vi "Process.vi"(7 "SubPnl Refnum":refnum<vi>, 8 "error in (no error)":errorcluster, 9 "Payload":string, 10 "Command":string, 11 "Core Class":refnum<class>) -> (0 "error out":errorcluster, 2 "Response":string, 3 "Match Present?":bool)   [LabVIEW 2019, in "MicronTemplateService.lvlib"]
uses:
  MicronTemplateService.lvlib
  <vilib>/LabJSON/Typedefs/Settings.ctl
  4e70540b-6f8f-44f3-a0e1-83e2859abde4.vi
  0b93bba3-7b7b-446a-8943-9293762f4055.vi
  2355c958-d1c3-4277-9a8a-c12bb77dc7b9.vi
  <vilib>/LabJSON/APIs/RunVIRefnum.vi
  <vilib>/JDP Science/JSONtext/Variant to JSON Text.vi
  <vilib>/JDP Science/JSONtext/support/Format JSON Object.vi
  <vilib>/JDP Science/JSONtext/LVClass Serializer/JSONtext LVClass Serializer.lvclass
  <vilib>/LabJSON/LabJSON.lvlib
  <vilib>/JDP Science/JSONtext/JSONtext.lvlib
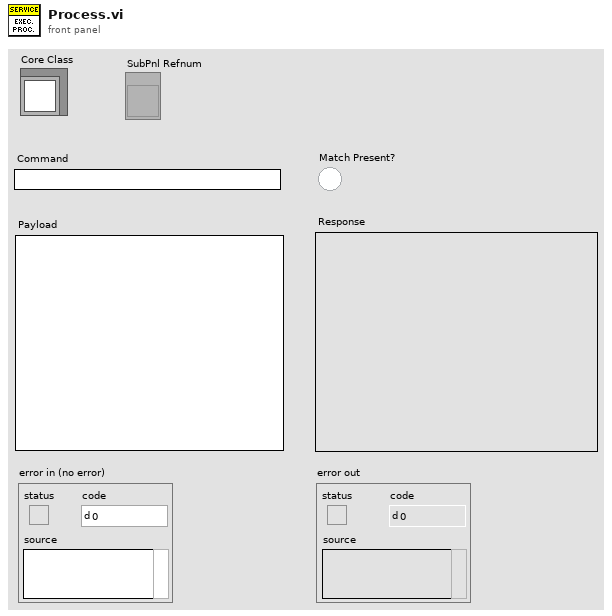
[diagram p1: front panel]
types:
  T1 = typedef "LabJSON.lvlib/Settings.ctl" = cluster{"Reinitialize to Default?":bool, "Show Front Panel?":bool, "Close Front Panel?":bool}
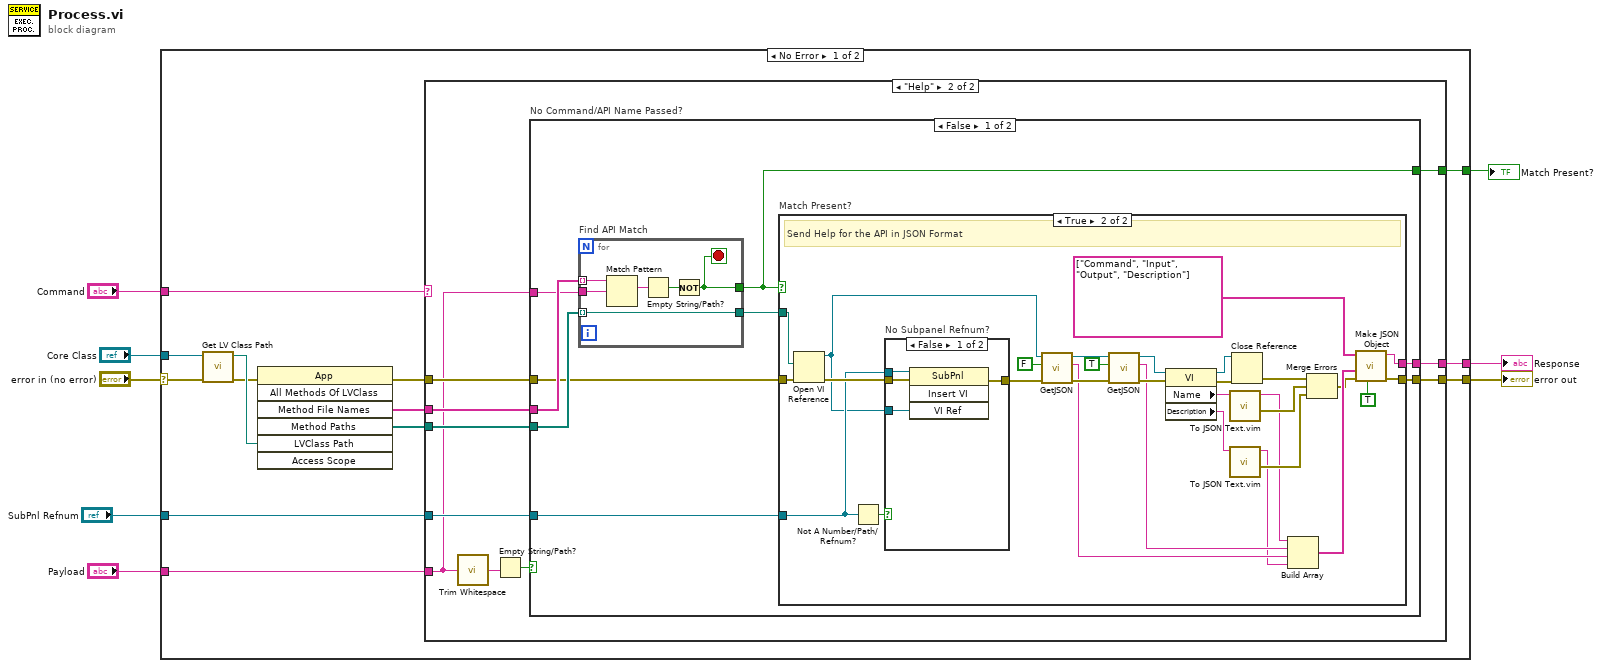
[diagram p0: block diagram]
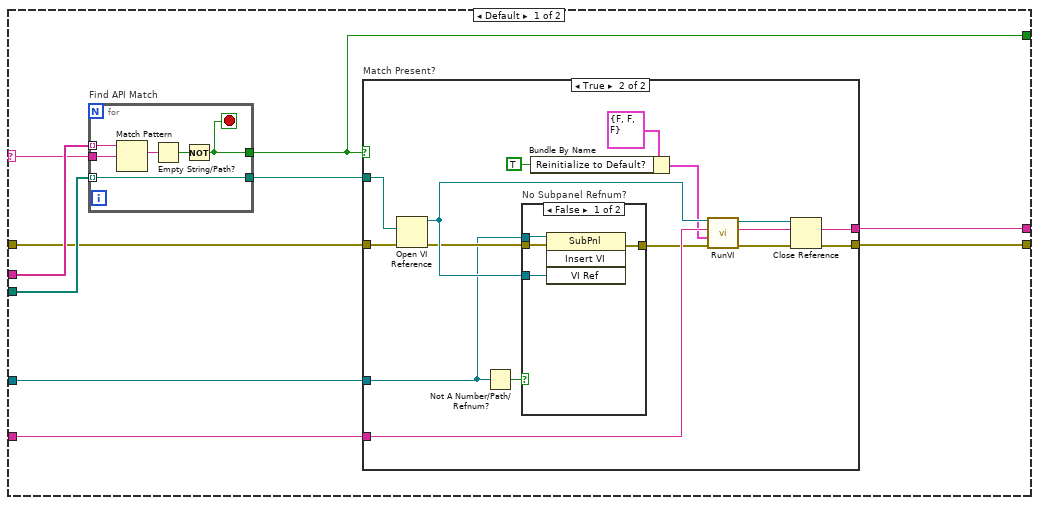
[diagram p2: hidden frame]
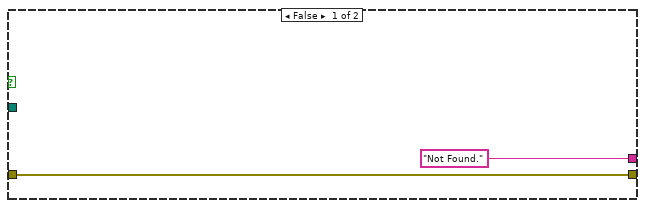
[diagram p5: hidden frame]
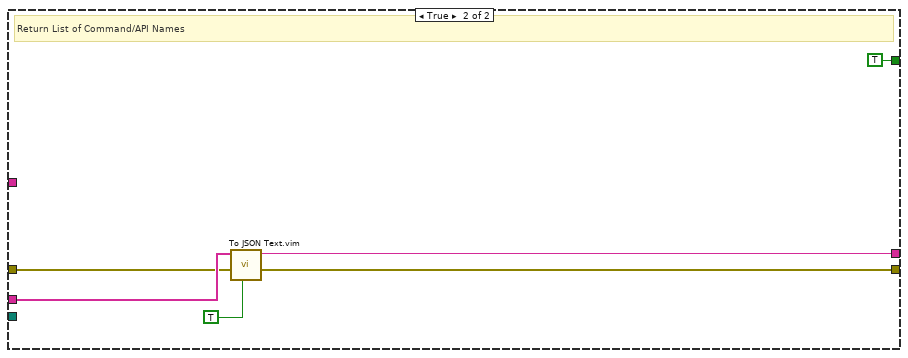
[diagram p7: hidden frame]
diagram:
  n1 = case shown="No Error" "error in (no error)" {
    selector: "error in (no error)" -> [w11 w127]
    tunnel: "Core Class" -> [w21 _]
    tunnel: "Command" -> [w17 _]
    tunnel: "Payload" -> [w16 _]
    tunnel: [w15 _] -> w5
    tunnel: "SubPnl Refnum" -> [w14 _]
    tunnel: [w10 w127] -> w2
    tunnel: [w9 _] -> w1
    frame No Error {
      n2 = call <vilib>:"Get LV Class Path.vi"("error in (no error)"=w11, "object"=w21) -> ("error out"=w13:errorcluster, "class path"=w20:path)  [unwired: 8 in]
      n3 = invoke class="App" method="All Methods Of LVClass"(error in=w13, "LVClass Path"=w20) -> (error out=w12:errorcluster, "Method File Names"=w19:string[], "Method Paths"=w18:path[])  [unwired: 5 in, 4 out]
      n4 = case shown="\"Help\"" w17 {
        selector: w17 -> [w29 _]
        tunnel: w19 -> [w31 w68]
        tunnel: w18 -> [w30 w67]
        tunnel: w16 -> [w28 w61]
        tunnel: [w27 w66] -> w15
        tunnel: w14 -> [w25 w65]
        tunnel: w12 -> [w24 w64]
        tunnel: [w23 w63] -> w10
        tunnel: [w22 w62] -> w9
        frame Default {
          n5 = for "Find API Match" {
            tunnel: w31 -> [w58] mode=indexing
            tunnel: w30 -> [w54] mode=indexing
            tunnel: w29 -> [w57]
            tunnel: [w54] -> w26
            tunnel: [w53] -> w22
            stop <- w53 stop-if-true
            n6 = Match Pattern(string=w58, regular expression=w57) -> (match substring=w56:string)  [unwired: 1 in, 3 out]
            n7 = Empty String/Path?(string/path=w56) -> (empty?=w55:bool)
            n8 = Not(x=w55) -> (.not. x?=w53:bool)
          }
          n9 = case "Match Present?" shown="True" w22 {
            tunnel: w28 -> [_ w47]
            tunnel: [_ w46] -> w27
            tunnel: w26 -> [_ w45]
            tunnel: w25 -> [_ w36]
            tunnel: w24 -> [w32 w40]
            tunnel: [w32 w34] -> w23
            frame False {
            }
            frame True {
              n10 = Open VI Reference(vi path=w45, error in (no error)=w40) -> (vi reference=w44:refnum<vi>, error out=w39:errorcluster)  [unwired: 4 in]
              n11 = Not A Number/Path/Refnum?(number/path/refnum=w36) -> (NaN/Path/Refnum?=w35:bool)
              n12 = case "No Subpanel Refnum?" shown="False" w35 {
                tunnel: w44 -> [w51 _]
                tunnel: w39 -> [w50 w52]
                tunnel: [w49 w52] -> w38
                tunnel: w36 -> [w48 _]
                frame False {
                  n13 = invoke class="SubPnl" method="Insert VI"(reference=w48, error in=w50, "VI Ref"=w51) -> (error out=w49:errorcluster)  [unwired: 1 in, 3 out]
                }
                frame True {
                }
              }
              n14 = Bundle By Name(cluster=T1 {"Reinitialize to Default?"=FALSE, "Show Front Panel?"=FALSE, "Close Front Panel?"=FALSE} ("Settings"), "Reinitialize to Default?"=TRUE) -> (w42:T1)
              n15 = call-poly <vilib>:"RunVI.vi"("Error In"=w38, "Settings"=w42, "JSON Input"=w47, "VI Refnum In"=w44) -> ("Error Out"=w37:errorcluster, "JSON Output"=w46:string, "VI Refnum Out"=w33:refnum<vi>)  [unwired: 5 in]
              n16 = Close Reference(reference=w33, error in (no error)=w37) -> (error out=w34:errorcluster)
            }
          }
        }
        frame "Help" {
          n17 = call <vilib>:"Trim Whitespace.vi"("string"=w61) -> ("trimmed string"=w60:string)  [unwired: 1 in]
          n18 = Empty String/Path?(string/path=w60) -> (empty?=w59:bool)
          n19 = case "No Command/API Name Passed?" shown="False" w59 {
            tunnel: w68 -> [w77 w126]
            tunnel: w67 -> [w76 _]
            tunnel: [w75 w122] -> w66
            tunnel: w65 -> [w73 _]
            tunnel: w64 -> [w72 w125]
            tunnel: [w71 w124] -> w63
            tunnel: [w70 TRUE] -> w62
            tunnel: w61 -> [w69 _]
            frame False {
              n20 = for "Find API Match" {
                tunnel: w77 -> [w120] mode=indexing
                tunnel: w76 -> [w116] mode=indexing
                tunnel: w69 -> [w119]
                tunnel: [w116] -> w74
                tunnel: [w115] -> w70
                stop <- w115 stop-if-true
                n21 = Match Pattern(string=w120, regular expression=w119) -> (match substring=w118:string)  [unwired: 1 in, 3 out]
                n22 = Empty String/Path?(string/path=w118) -> (empty?=w117:bool)
                n23 = Not(x=w117) -> (.not. x?=w115:bool)
              }
              n24 = case "Match Present?" shown="True" w70 {
                tunnel: ["Not Found." ("JSON Output") w97] -> w75
                tunnel: w74 -> [_ w109]
                tunnel: w73 -> [_ w106]
                tunnel: w72 -> [w79 w108]
                tunnel: [w79 w99] -> w71
                frame False {
                }
                frame True {
                  # "Send Help for the API in JSON Format"
                  n25 = Open VI Reference(vi path=w109, error in (no error)=w108) -> (vi reference=w103:refnum<vi>, error out=w107:errorcluster)  [unwired: 4 in]
                  n26 = Not A Number/Path/Refnum?(number/path/refnum=w106) -> (NaN/Path/Refnum?=w105:bool)
                  n27 = case "No Subpanel Refnum?" shown="False" w105 {
                    tunnel: w103 -> [w113 _]
                    tunnel: w107 -> [w112 w114]
                    tunnel: [w111 w114] -> w104
                    tunnel: w106 -> [w110 _]
                    frame False {
                      n28 = invoke class="SubPnl" method="Insert VI"(reference=w110, error in=w112, "VI Ref"=w113) -> (error out=w111:errorcluster)  [unwired: 1 in, 3 out]
                    }
                    frame True {
                    }
                  }
                  n29 = call <vilib>:"GetJSON.vi"("Error In"=w104, "Controls?"=FALSE, "VI Refnum In"=w103) -> ("Error Out"=w93:errorcluster, "JSON Out"=w87:string, "VI Refnum Out"=w91:refnum<vi>)  [unwired: 6 in]
                  n30 = call <vilib>:"GetJSON.vi"("Error In"=w93, "Controls?"=TRUE, "VI Refnum In"=w91) -> ("Error Out"=w92:errorcluster, "JSON Out"=w88:string, "VI Refnum Out"=w89:refnum<vi>)  [unwired: 6 in]
                  n31 = property class="VI"(reference=w89, error in=w92) -> (reference out=w100:refnum<vi>, error out=w101:errorcluster, "Name"=w86:string, "Description"=w85:string)
                  n32 = call "To JSON Text.vim"("Anything"=w86) -> ("error out"=w83:errorcluster, "<JSON>"=w81:string)  [unwired: 9 in]
                  n33 = call "To JSON Text.vim"("Anything"=w85) -> ("error out"=w82:errorcluster, "<JSON>"=w80:string)  [unwired: 9 in]
                  n34 = Close Reference(reference=w100, error in (no error)=w101) -> (error out=w96:errorcluster)
                  n35 = Build Array(w81, w88, w87, w80) -> (w95:string[])
                  n36 = Merge Errors(w96, w83, w82) -> (w84:errorcluster)
                  n37 = call <vilib>:"Make JSON Object.vi"("Pretty Print?"=TRUE, "error in (no error)"=w84, "JSON Items"=w95, "Item Names"=string[] ["Command", "Input", "Output", "Description"]) -> ("error out"=w99:errorcluster, "<JSON>"=w97:string)  [unwired: 6 in]
                }
              }
            }
            frame True {
              # "Return List of Command/API Names"
              n38 = call "To JSON Text.vim"("Pretty Print?"=TRUE, "error in (no error)"=w125, "Anything"=w126) -> ("error out"=w124:errorcluster, "<JSON>"=w122:string)  [unwired: 7 in]
            }
          }
        }
      }
    }
    frame Error {
    }
  }
  "Response" <- w5
  "error out" <- w2
  "Match Present?" <- w1
